vi "fixConnect4Array.vi"(11 "AllObjs[]":refnum<vi>[](array[refnum])) -> (3 "Array":refnum<vi>[](array[refnum]))   [LabVIEW 2014]
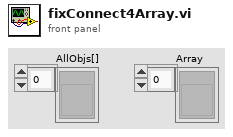
[diagram p1: front panel]
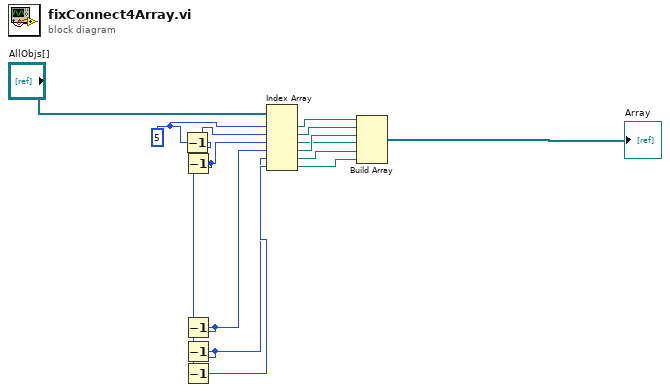
[diagram p0: block diagram]
diagram:
  w6 = 5
  n1 = Decrement(x=w6) -> (x-1=w4:i32)
  n2 = Decrement(x=w4) -> (x-1=w3:i32)
  n3 = Decrement(x=w3) -> (x-1=w2:i32)
  n4 = Decrement(x=w2) -> (x-1=w1:i32)
  n5 = Decrement(x=w1) -> (x-1=w5:i32)
  n6 = Index Array(array="AllObjs[]", index #1=w6, index #2=w4, index #3=w3, index #4=w2, index #5=w1, index #6=w5) -> (element #1=w8:refnum<vi>, element #2=w9:refnum<vi>, element #3=w10:refnum<vi>, element #4=w11:refnum<vi>, element #5=w12:refnum<vi>, element #6=w13:refnum<vi>)
  n7 = Build Array(w8, w9, w11, w10, w12, w13) -> (→"Array":refnum<vi>[])
